vi "DAQmx Create Channel (TEDS-AI-Voltage-Custom with Excitation).vi"(0 "task in":refnum<k21>, 1 "maximum value":dbl=10.0 format="%0.2f", 2 "minimum value":dbl=-10.0 format="%0.2f", 3 "input terminal configuration":i32(ring)=-1 items=["default"=-1, "RSE"=10083, "NRSE"=10078, "Differential"=10106, "Pseudodifferential"=12529], 5 "physical channels":tag, 7 "name to assign":string, 9 "units":i32(ring)=12516 items=["From TEDS"=12516, "From Custom Scale"=10065], 10 "voltage excitation value":dbl format="%.6f", 11 "error in":errorcluster, 12 "custom scale name":tag, 13 "voltage excitation source":i32(ring)=10200 items=["Internal"=10200, "External"=10167, "None"=10230]) -> (4 "task out":refnum<k21>, 15 "error out":errorcluster)   [LabVIEW 2011]
doc: "Creates channel(s) to measure voltage. Use this instance for custom sensors that require excitation. You can use the excitation to scale the measurement. You must configure the physical channel(s) with TEDS information to use this VI."
uses:
  C:/Program Files/National Instruments/LabVIEW 2011/resource/objmgr/daqmx.rc
panel:
  # "input limits"
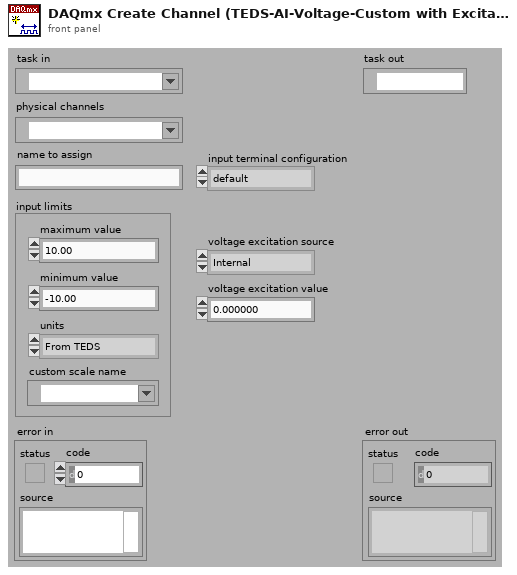
[diagram p1: front panel]
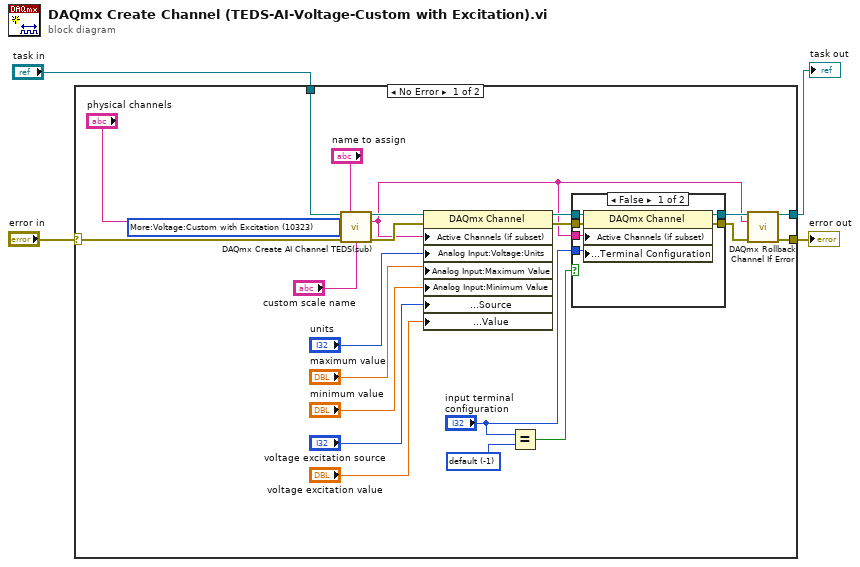
[diagram p0: block diagram]
diagram:
  n1 = case shown="No Error" "error in" {
    selector: "error in" -> [w26 w36]
    tunnel: [w8 w36] -> w4
    tunnel: "task in" -> [w27 w37]
    tunnel: [w7 w37] -> w1
    frame No Error {
      w5 = 10323 items=["Voltage"=10322, "Current"=10134, "More:Voltage:Custom with Excitation"=10323, "More:Current:Custom with Excitation"=10136, "Frequency"=10181, "Period"=10257, "Resistance"=10278, "Temperature:Thermocouple"=10303, "Temperature:Thermistor"=10302, "Temperature:RTD"=10301, "Temperature:Built-in Sensor"=10311, "Strain Gage"=10300, "LVDT"=10352, "RVDT"=10353, "Accelerometer:Voltage Input"=10355, "Accelerometer:Current Input"=10356, "Sound Pressure:Microphone"=10354, "TEDS"=12531] ("measurement type")
      w13 = -1 items=["default"=-1, "differential"=10106, "RSE"=10083, "NRSE"=10078] ("input terminal configuration")
      n2 = call "DAQmx Create AI Channel TEDS(sub).vi"("task in"=w27, "virtual channel name"="name to assign", "physical channel name"="physical channels", "measurement type"=w5, "error in"=w26, "custom scale"="custom scale name") -> ("task out"=w11:refnum<k21>, "channel names"=w6:string, "error out"=w24:errorcluster)  [unwired: 7 out]
      n3 = property class="DAQmx Channel"(reference=w11, error in=w24, "Active Channels (if subset)"=w6, "Analog Input:Voltage:Units"="units", "Analog Input:Maximum Value"="maximum value", "Analog Input:Minimum Value"="minimum value", "Analog Input:General Properties:Signal Conditioning:Excitation:Source"="voltage excitation source", "Analog Input:General Properties:Signal Conditioning:Excitation:Value"="voltage excitation value") -> (reference out=w19:refnum<k21>, error out=w18:errorcluster)
      n4 = Equal?(x="input terminal configuration", y=w13) -> (x = y?=w20:bool)
      n5 = case shown="False" w20 {
        tunnel: "input terminal configuration" -> [w30 _]
        tunnel: w19 -> [w28 w35]
        tunnel: w18 -> [w33 w34]
        tunnel: [w32 w35] -> w10
        tunnel: [w31 w34] -> w9
        tunnel: w6 -> [w29 _]
        frame False {
          n6 = property class="DAQmx Channel"(reference=w28, error in=w33, "Active Channels (if subset)"=w29, "Analog Input:General Properties:Input Configuration:Terminal Configuration"=w30) -> (reference out=w32:refnum<k21>, error out=w31:errorcluster)
        }
        frame True {
        }
      }
      n7 = call "DAQmx Rollback Channel If Error.vi"("task in"=w10, "channel names"=w6, "error in"=w9) -> ("task out"=w7:refnum<k21>, "error out"=w8:errorcluster)  [unwired: 11 out]
    }
    frame Error {
    }
  }
  "error out" <- w4
  "task out" <- w1
